vi "mean.vi"(9 "Numeric 2":sgl, 10 "n":i32, 11 "Numeric":sgl) -> (2 "mean":sgl)   [LabVIEW 2015]
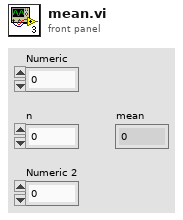
[diagram p1: front panel]
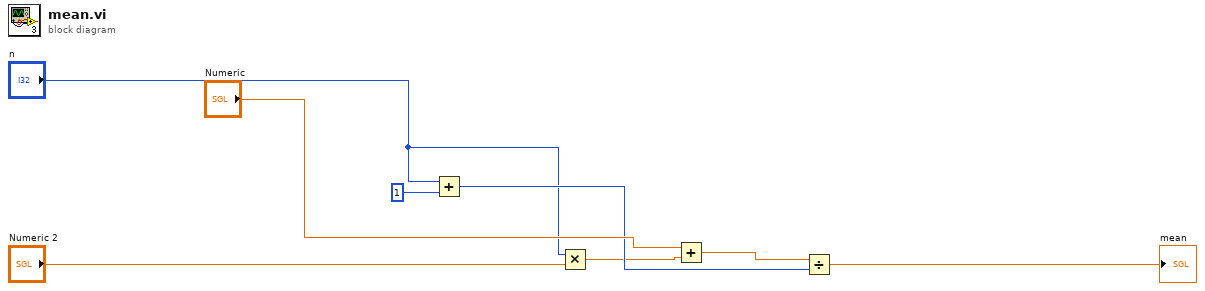
[diagram p0: block diagram]
diagram:
  n1 = Add(x="n", y=1) -> (x+y=w7:i32)
  n2 = Multiply(x="n", y="Numeric 2") -> (x*y=w3:sgl)
  n3 = Add(x="Numeric", y=w3) -> (x+y=w4:sgl)
  n4 = Divide(x=w4, y=w7) -> (x/y=→"mean":sgl)
